vi "db_term.vi"(0 "REFERENCE IN":T1, 5 "ERROR IN":errorcluster) -> (19 "ERROR OUT":errorcluster)   [LabVIEW 2018, in "db_lib R3.lvlib"]
uses:
  db_lib R3.lvlib
  <vilib>/addons/database/Connection.llb/Conn ObjectReference.ctl
  <vilib>/addons/database/NI_Database_API.lvlib
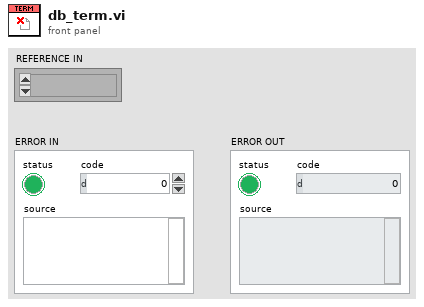
[diagram p1: front panel]
types:
  T1 = typedef "NI_Database_API.lvlib/Conn ObjectReference.ctl" = refnum<k1>
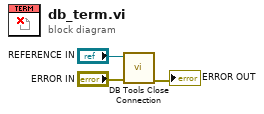
[diagram p0: block diagram]
diagram:
  n1 = call <vilib>:"DB Tools Close Connection.vi"("error in (no error)"="ERROR IN", "connection reference"="REFERENCE IN") -> ("error out"=→"ERROR OUT":errorcluster)  [unwired: 5 in]
